vi "DIO write.vi"(0 "FPGA VI Reference In":refnum<k20>, 5 "Timing data":u64[](array[numeric]), 7 "Outputs of port A and B":u64[](array[numeric]), 9 "Outputs of port C and D":u64[](array[numeric]), 11 "error in":errorcluster) -> (4 "FPGA VI Reference Out":refnum<k20>, 15 "error out":errorcluster)   [LabVIEW 2017]
uses:
  <vilib>/Utility/error.llb/Error Cluster From Error Code.vi
  <vilib>/rvi/errors/niLvFpgaAdjustHostInterfaceError.vi
  <vilib>/rvi/interface/nirviMethod/nirviMethod.xnode
  <vilib>/FPGAPlugInAG/Dynamic/niLvFpga_WriteFifo_Dynamic.vi
  <vilib>/rvi/errors/niLvFpgaMergeErrorWithErrorCode.vi
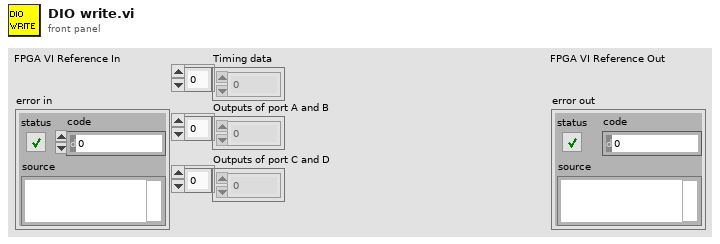
[diagram p1: front panel]
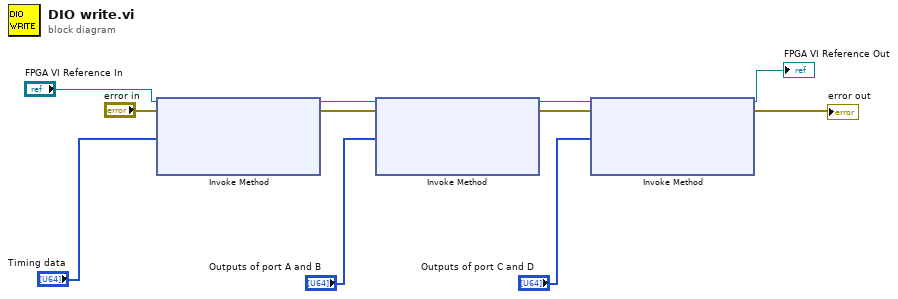
[diagram p0: block diagram]
diagram:
  n1 = xnode "Invoke Method"("FPGA VI Reference In"="FPGA VI Reference In", "error in"="error in", "Data"="Timing data") -> ("FPGA VI Reference Out"=w10:refnum<k20>, "error out"=w8:errorcluster)  [unwired: 1 in, 1 out]
  n2 = xnode "Invoke Method"("FPGA VI Reference In"=w10, "error in"=w8, "Data"="Outputs of port A and B") -> ("FPGA VI Reference Out"=w7:refnum<k20>, "error out"=w6:errorcluster)  [unwired: 1 in, 1 out]
  n3 = xnode "Invoke Method"("FPGA VI Reference In"=w7, "error in"=w6, "Data"="Outputs of port C and D") -> ("FPGA VI Reference Out"=→"FPGA VI Reference Out":refnum<k20>, "error out"=→"error out":errorcluster)  [unwired: 1 in, 1 out]
